vi "Acq Reset.vi"(0 "fpga reference in":refnum<k20>, 5 "reset dsp":bool, 7 "reset stream control":bool, 9 "reset waveform streaming":bool, 11 "error in (no error)":errorcluster) -> (4 "fpga reference out":refnum<k20>, 15 "error out":errorcluster)   [LabVIEW 2021, in "Digitizer Control.lvclass"]
doc: "Resets the selected blocks in the acquisition path.\n\nInputs:\n\n<B>fpga reference in</B>: Reference to the FPGA target.\n\n<B>reset dsp</B>: A true on this input resets the DSP chain in the acquisition path.\n\n<B>reset stream control</B>: A true on this input resets the acquisition stream control.\n\n<B>reset waveform streaming</B>: A true on this input resets the waveform streaming.\n\nOutput:\n\n<B>fpga reference out</B>: The reference passed on the <B>fpga reference in</B> input."
uses:
  Digitizer Control.lvclass
  <vilib>/Utility/error.llb/Error Cluster From Error Code.vi
  <vilib>/rvi/errors/niLvFpgaAdjustHostInterfaceError.vi
  <vilib>/rvi/interface/nirviReadWriteControl/nirviReadWriteControl.xnode
  <vilib>/ErrorRing/Error Ring.xnode
  NiFpgaLv.dll
  <vilib>/rvi/interface/Simulation/niFpgaSimulationCallBeginRW.vi
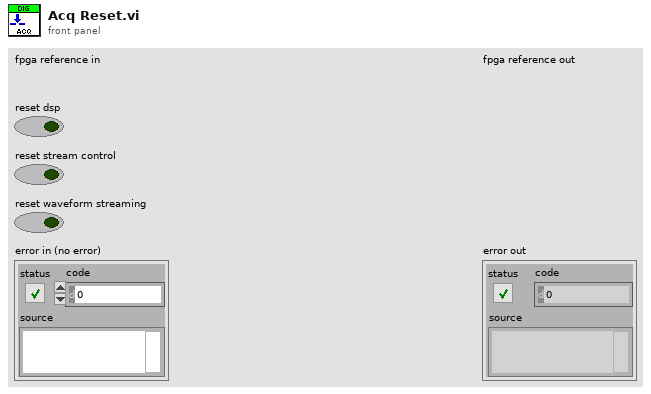
[diagram p1: front panel]
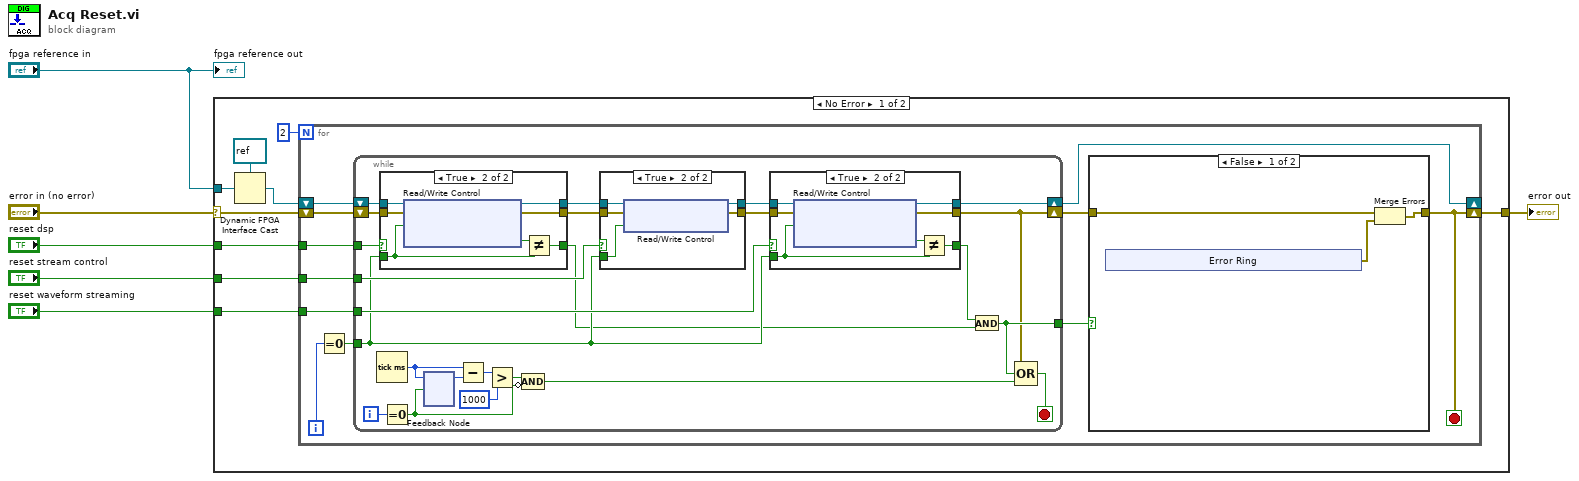
[diagram p0: block diagram]
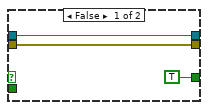
[diagram p3: hidden frame]
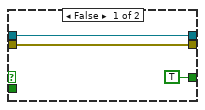
[diagram p5: hidden frame]
diagram:
  n1 = case shown="No Error" "error in (no error)" {
    selector: "error in (no error)" -> [w10 w87]
    tunnel: "fpga reference in" -> [w12 _]
    tunnel: [w11 w87] -> w5
    tunnel: "reset dsp" -> [w9 _]
    tunnel: "reset stream control" -> [w8 _]
    tunnel: "reset waveform streaming" -> [w7 _]
    frame No Error {
      n2 = Dynamic FPGA Interface Cast(Session In=refnum<k20> refnum ("FPGA Interface"), Type=w12) -> (Session Out=w13:refnum<k20>)
      n3 = for {
        N: 2 -> [_]
        shift-right: [w16] -> w11
        shift-left: w10 -> [w26]
        shift-right: [w23] -> _
        shift-left: w13 -> [w25]
        tunnel: w9 -> [w20]
        tunnel: w8 -> [w19]
        tunnel: w7 -> [w18]
        i -> [w17]
        stop <- w16 stop-if-true
        n4 = Equal To 0?(x=w17) -> (x = 0?=w21:bool)
        n5 = while {
          shift-right: [w38] -> w23
          shift-left: w25 -> [w59]
          shift-right: [w39] -> w24
          shift-left: w26 -> [w58]
          tunnel: [w40] -> w22
          tunnel: w21 -> [w43]
          tunnel: w20 -> [w50]
          tunnel: w19 -> [w47]
          tunnel: w18 -> [w44]
          i -> [w37]
          stop <- w36 stop-if-true
          n6 = Tick Count (ms)() -> (millisecond timer value=w57:u32)
          n7 = case shown="True" w50 {
            tunnel: w59 -> [w79 w86]
            tunnel: w58 -> [w78 w85]
            tunnel: [w79 w84] -> w48
            tunnel: [w78 w83] -> w49
            tunnel: w43 -> [_ w81]
            tunnel: [TRUE w80] -> w41
            frame False {
            }
            frame True {
              n8 = xnode "Read/Write Control"("FPGA VI Reference In"=w86, "error in"=w85, "acq.dsp.reset"=w81) -> ("FPGA VI Reference Out"=w84:refnum<k20>, "error out"=w83:errorcluster, "acq.dsp.reset done"=w82:bool)
              n9 = Not Equal?(x=w82, y=w81) -> (x != y?=w80:bool)
            }
          }
          n10 = Equal To 0?(x=w37) -> (x = 0?=w52:bool)
          n11 = feedback-in #1(w57, w52) -> ()
          n12 = feedback #1() -> (w56:u32)  [unwired: 1 in]
          n13 = Subtract(x=w57, y=w56) -> (x-y=w55:u32)
          n14 = Greater?(x=w55, y=u32 1000) -> (0:w53:bool)
          n15 = Compound Arithmetic op=AND(w53, invert w52) -> (w51:bool)
          n16 = case shown="True" w47 {
            tunnel: w48 -> [w71 w76]
            tunnel: w49 -> [w70 w75]
            tunnel: [w71 w74] -> w45
            tunnel: [w70 w73] -> w46
            tunnel: w43 -> [_ w72]
            frame False {
            }
            frame True {
              n17 = xnode "Read/Write Control"("FPGA VI Reference In"=w76, "error in"=w75, "acq.stream.reset"=w72) -> ("FPGA VI Reference Out"=w74:refnum<k20>, "error out"=w73:errorcluster)
            }
          }
          n18 = case shown="True" w44 {
            tunnel: w45 -> [w62 w69]
            tunnel: w46 -> [w61 w68]
            tunnel: [w62 w67] -> w38
            tunnel: [w61 w66] -> w39
            tunnel: w43 -> [_ w64]
            tunnel: [TRUE w63] -> w42
            frame False {
            }
            frame True {
              n19 = xnode "Read/Write Control"("FPGA VI Reference In"=w69, "error in"=w68, "acq.wfm.reset"=w64) -> ("FPGA VI Reference Out"=w67:refnum<k20>, "error out"=w66:errorcluster, "acq.wfm.reset done"=w65:bool)
              n20 = Not Equal?(x=w65, y=w64) -> (x != y?=w63:bool)
            }
          }
          n21 = And(x=w42, y=w41) -> (x .and. y?=w40:bool)
          n22 = Compound Arithmetic op=OR(w39, w40, w51) -> (w36:bool)
        }
        n23 = case shown="False" w22 {
          tunnel: w24 -> [w29 w35]
          tunnel: [w27 w35] -> w16
          frame False {
            n24 = xnode "Error Ring"() -> ("error out"=w28:errorcluster)
            n25 = Merge Errors(w29, w28) -> (w27:errorcluster)
          }
          frame True {
          }
        }
      }
    }
    frame Error {
    }
  }
  "error out" <- w5
  "fpga reference out" <- "fpga reference in"
